vi "Spectrum Recorder.vi"() -> ()   [LabVIEW 2016]
uses:
  Spectrum Recorder Configuration.ctl
  Spectrum Recorder.lvclass
  Spectrum Recorder.lvclass/Spectrum Recorder.ctl
  <vilib>/ActorFramework/Message Enqueuer/Message Enqueuer.lvclass/Message Enqueuer.ctl
  Write Phase.vi
  Write Data file path indicator ref.vi
  Write State ref.vi
  Write Spectrum graph ref.vi
  Write Address.vi
  <vilib>/ActorFramework/Message Enqueuer/Enqueue.vi
  <vilib>/ActorFramework/Stop Msg/Stop Msg.lvclass
  D:/Program Files/National Instruments/LabVIEW 2016/vi.lib/ActorFramework/Message/Message.lvclass
  Write Spectrum Recorder Configuration.vi
  <vilib>/ActorFramework/Message Priority Queue/Priority Enqueue.vi
  <vilib>/ErrorRing/Error Ring.xnode
panel:
  in  "Address":string="192.168.1.100"
  in  "Phase":dbl(slide) scale=-180.0..180.0
  in  "Open digitizer":bool
  out "State":bool
  out "Data file path":path=path "C:/Data"
  in  "Exit":bool
  in  "Stop":bool
  in  "Record":bool
  in  "Configuration":T1={"Start"=500000.0, "End"=2000000.0, "Duration"=40.0, "Filter time constant"=0.004, "Repeat (-1: forever)"=1, "Update rate"=1.0, "Data storage folder"=path "C:/Data"} {"Update rate" min=0.001 max=10.0 step=0.001 format="%#_6ps"; "Repeat (-1: forever)" format="%.0p"; "Filter time constant" format="%#_6ps"; "Duration" format="%#_6ps"; "End" format="%#_6pHz"; "Start" format="%#_6pHz"}
  out "Spectrum plot":cluster{dbl[], dbl[]}[](graph)
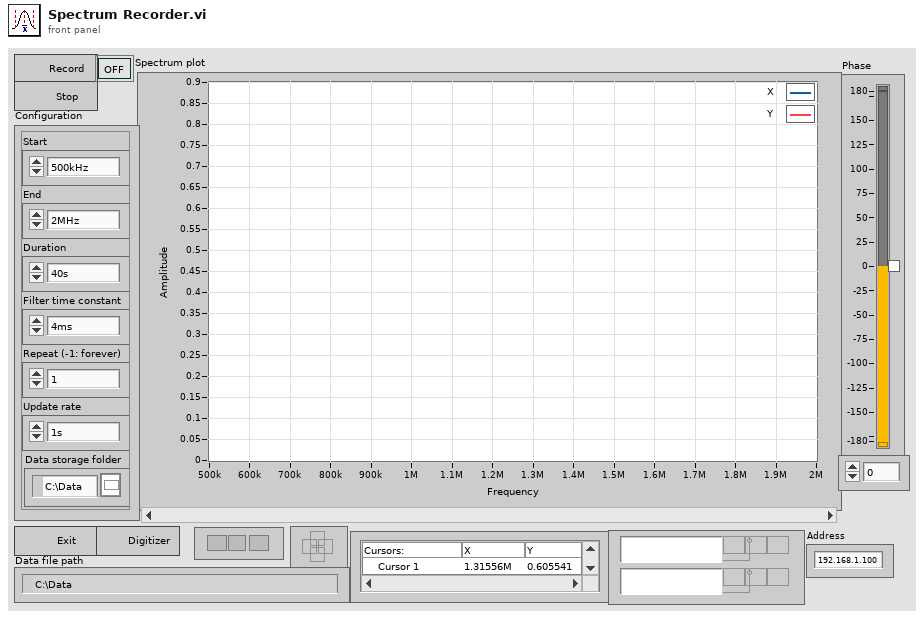
[diagram p1: front panel]
types:
  T1 = typedef "Spectrum Recorder Configuration.ctl" = cluster{"Start":dbl, "End":dbl, "Duration":dbl, "Filter time constant":dbl, "Repeat (-1: forever)":i32, "Update rate":dbl, "Data storage folder":path}
  T2 = enum32{"invalid app kind", "Development System", "Run Time System", "Student Edition", "Embedded LabVIEW", "Evaluation", "Custom"}
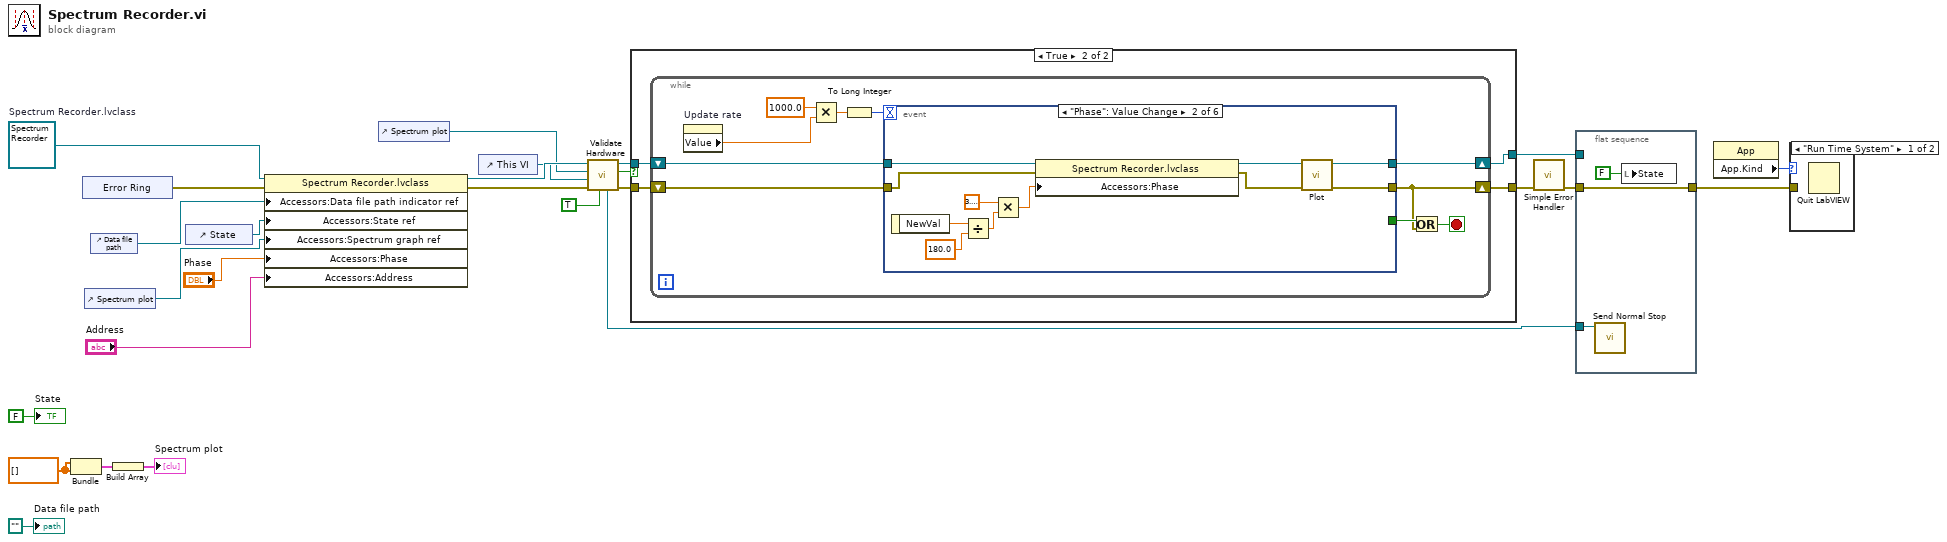
[diagram p0: block diagram]
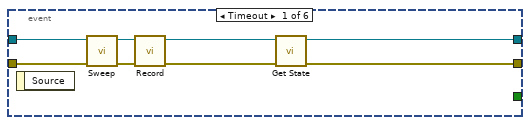
[diagram p4: hidden frame]
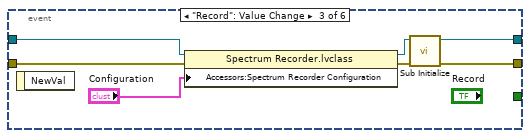
[diagram p5: hidden frame]
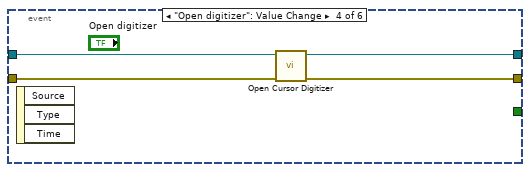
[diagram p6: hidden frame]
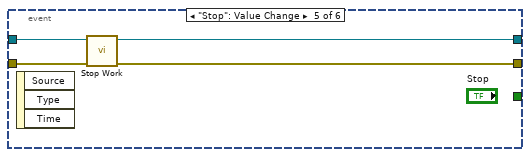
[diagram p7: hidden frame]
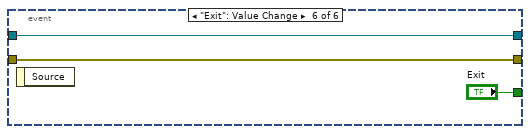
[diagram p8: hidden frame]
diagram:
  w23 = dbl[] []
  w15 = refnum<class "Spectrum Recorder.lvclass"> refnum  # Spectrum Recorder.lvclass
  n1 = Bundle(w23, w23) -> (w22:cluster{dbl[], dbl[]})  [unwired: 1 in]
  n2 = xnode "Error Ring"() -> ("error out"=w26:errorcluster)
  n3 = control-ref of="Spectrum plot"() -> (w20:refnum<vi>)
  n4 = control-ref of="Data file path"() -> (w25:refnum<vi>)
  n5 = Build Array(w22) -> (→"Spectrum plot":cluster{dbl[], dbl[]}[])
  n6 = control-ref of="State"() -> (w24:refnum<vi>)
  n7 = property class="Spectrum Recorder.lvclass"(reference=w15, error in=w26, "Accessors:Data file path indicator ref"=w25, "Accessors:State ref"=w24, "Accessors:Spectrum graph ref"=w20, "Accessors:Phase"="Phase", "Accessors:Address"="Address") -> (reference out=w14:refnum<class "Spectrum Recorder.lvclass">, error out=w12:errorcluster)
  n8 = control-ref of="Spectrum plot"() -> (w6:refnum<vi>)
  n9 = control-ref of="This VI"() -> (w4:refnum<vi>)
  n10 = call-dynamic "Validate Hardware.vi"("Interactive"=TRUE, "error in (no error)"=w12, "Pane"=w4, "XY graph ref"=w6, "Spectrum Recorder in"=w14) -> ("error out"=w11:errorcluster, "Valid"=w10:bool, "Spectrum Recorder out"=w13:refnum<class "Spectrum Recorder.lvclass">, "Actor's Enqueuer"=w3:refnum<class "Message Enqueuer.lvclass">)  [unwired: 3 in]
  n11 = case shown="True" w10 {
    tunnel: w11 -> [w28 w32]
    tunnel: w13 -> [w27 w31]
    tunnel: [w28 w30] -> w19
    tunnel: [w27 w29] -> w5
    frame False {
    }
    frame True {
      n12 = while {
        shift-right: [w38] -> w29
        shift-left: w31 -> [w39]
        shift-right: [w35] -> w30
        shift-left: w32 -> [w37]
        stop <- w36 stop-if-true
        n13 = property on="Update rate" class="DigNum (strict)"() -> ("Value"=w33:dbl)  [unwired: 2 in, 2 out]
        n14 = Multiply(x=1000.0 ("y"), y=w33) -> (x*y=w41:dbl)
        n15 = To Long Integer(number=w41) -> (32bit integer=w40:i32)
        n16 = event shown="[1] \"Phase\": Value Change" {
          selector: _ -> [_ _ _ _ _ _]
          dyn-events: _ -> [_ _ _ _ _ _]
          timeout: w40 -> [_ _ _ _ _ _]
          tunnel: [_ _ _ _ _ "Exit"] -> w42
          tunnel: w39 -> [w48 w61 w64 w70 w75 w78]
          tunnel: [w43 w59 w66 w69 w73 w78] -> w38
          tunnel: w37 -> [w50 w56 w68 w72 w76 w77]
          tunnel: [w45 w58 w67 w71 w74 w77] -> w35
          event Timeout {
            n17 = event-data() -> ()  [unwired: 1 in, 1 out]
            n18 = call-dynamic "Sweep.vi"("error in (no error)"=w50, "Spectrum Recorder in"=w48) -> ("error out"=w49:errorcluster, "Spectrum Recorder out"=w46:refnum<class "Spectrum Recorder.lvclass">)  [unwired: 8 in]
            n19 = call-dynamic "Record.vi"("error in (no error)"=w49, "Spectrum Recorder in"=w46) -> ("error out"=w47:errorcluster, "Spectrum Recorder out"=w44:refnum<class "Spectrum Recorder.lvclass">)  [unwired: 8 in]
            n20 = call-dynamic "Get State.vi"("error in (no error)"=w47, "Spectrum Recorder in"=w44) -> ("error out"=w45:errorcluster, "Spectrum Recorder out"=w43:refnum<class "Spectrum Recorder.lvclass">)  [unwired: 6 in, 2 out]
          }
          event "Phase": Value Change {
            n21 = event-data() -> ("NewVal"=w57:dbl)  [unwired: 1 in]
            n22 = Divide(x=w57, y=180.0) -> (x/y=w54:dbl)
            n23 = Multiply(x=3.141592653589793, y=w54) -> (x*y=w52:dbl)
            n24 = property class="Spectrum Recorder.lvclass"(reference=w61, error in=w56, "Accessors:Phase"=w52) -> (reference out=w60:refnum<class "Spectrum Recorder.lvclass">, error out=w55:errorcluster)
            n25 = call-dynamic "Plot.vi"("error in (no error)"=w55, "Spectrum Recorder in"=w60) -> ("error out"=w58:errorcluster, "Spectrum Recorder out"=w59:refnum<class "Spectrum Recorder.lvclass">)  [unwired: 8 in]
          }
          event "Record": Value Change {
            n26 = event-data() -> ()  [unwired: 1 in, 1 out]
            n27 = property class="Spectrum Recorder.lvclass"(reference=w64, error in=w68, "Accessors:Spectrum Recorder Configuration"="Configuration") -> (reference out=w63:refnum<class "Spectrum Recorder.lvclass">, error out=w65:errorcluster)
            n28 = call-dynamic "Sub Initialize.vi"("error in (no error)"=w65, "Spectrum Recorder in"=w63) -> ("error out"=w67:errorcluster, "Spectrum Recorder out"=w66:refnum<class "Spectrum Recorder.lvclass">)  [unwired: 7 in, 1 out]
          }
          event "Open digitizer": Value Change {
            n29 = event-data() -> ()  [unwired: 1 in, 3 out]
            n30 = call-dynamic "Open Cursor Digitizer.vi"("error in (no error)"=w72, "Spectrum Recorder in"=w70) -> ("error out"=w71:errorcluster, "Spectrum Recorder out"=w69:refnum<class "Spectrum Recorder.lvclass">)  [unwired: 8 in]
          }
          event "Stop": Value Change {
            n31 = event-data() -> ()  [unwired: 1 in, 3 out]
            n32 = call-dynamic "Stop Work.vi"("error in (no error)"=w76, "Spectrum Recorder in"=w75) -> ("error out"=w74:errorcluster, "Spectrum Recorder out"=w73:refnum<class "Spectrum Recorder.lvclass">)  [unwired: 8 in]
          }
          event "Exit": Value Change {
            n33 = event-data() -> ()  [unwired: 1 in, 1 out]
          }
        }
        n34 = Or(x=w42, y=w35) -> (x .or. y?=w36:bool)
      }
    }
  }
  n35 = call <vilib>:"Simple Error Handler.vi"("error in (no error)"=w19) -> ("error out"=w16:errorcluster)  [unwired: 4 in, 4 out]
  n36 = flat-sequence {
    tunnel: w16 -> [w81]
    tunnel: [w81] -> w7
    tunnel: w5 -> [_]
    tunnel: w3 -> [w80]
    frame #0 {
      n37 = call <vilib>:"Send Normal Stop.vi"("Message Enqueuer"=w80) -> ()  [unwired: 10 in, 1 out]
      n38 = local write "State"(FALSE ("State")) -> ()
    }
  }
  n39 = property class="App"() -> ("App.Kind"=w8:T2)  [unwired: 2 in, 2 out]
  n40 = case shown="\"Run Time System\"" w8 {
    tunnel: w7 -> [_ _]
    frame "Run Time System" {
      n41 = Quit LabVIEW() -> ()  [unwired: 1 in]
    }
    frame "Development System", Default {
    }
  }
  "Data file path" <- path ""
  "State" <- FALSE ("State")
